vi "Example1.vi"() -> (0 "error out":errorcluster)   [LabVIEW 2020, in "Clippy.lvclass"]
uses:
  Clippy.lvclass
  AnimationTypes.ctl
panel:
  in  "Question":string
  out "Answer":string
  out "Picture":picture
  in  "Animate":bool
  in  "Animation":T1
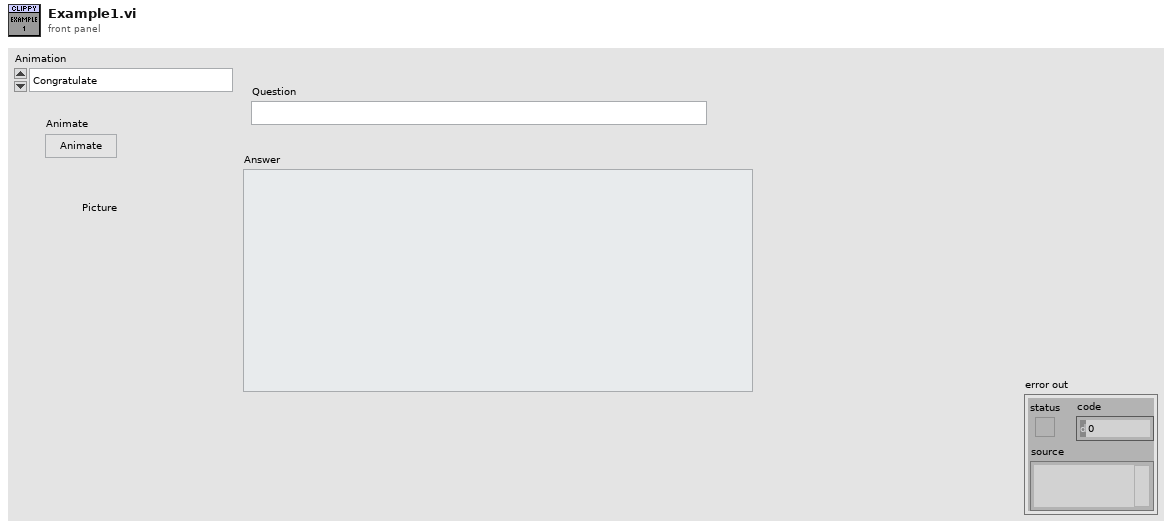
[diagram p1: front panel]
types:
  T1 = typedef "Clippy.lvclass/AnimationTypes.ctl" = enum16{"Congratulate", "LookRight", "SendMail", "Thinking", "Explain", "IdleRopePile", "IdleAtom", "Print", "Hide", "GetAttention", "Save", "GetTechy", "GestureUp", "Idle1_1", "Processing", "Alert", "LookUpRight", "IdleSideToSide", "GoodBye", "LookLeft", "IdleHeadScratch", "LookUpLeft", "CheckingSomething", "Hearing_1", "GetWizardy", "IdleFingerTap", "GestureLeft", "Wave", "GestureRight", "Writing", "IdleSnooze", "LookDownRight", "GetArtsy", "Show", "LookDown", "Searching", "EmptyTrash", "Greeting", "LookUp", "GestureDown", "RestPose", "IdleEyeBrowRaise", "LookDownLeft"}
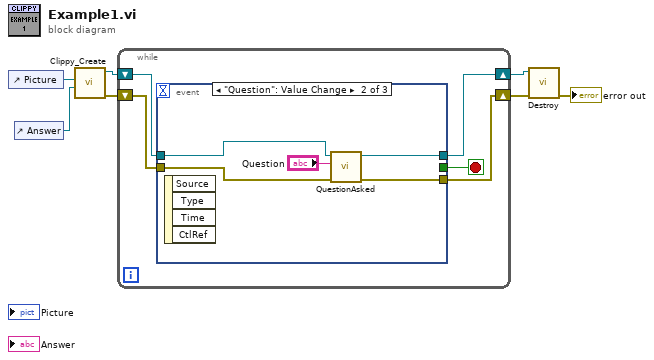
[diagram p0: block diagram]
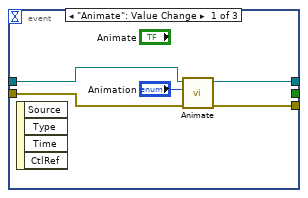
[diagram p2: hidden frame]
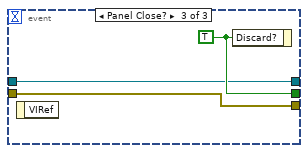
[diagram p3: hidden frame]
diagram:
  n1 = control-ref of="Picture"() -> (w2:refnum<vi>)
  n2 = control-ref of="Answer"() -> (w1:refnum<vi>)
  n3 = call "Clippy_Create.vi"("AnswerRef"=w1, "ClippyPictureRef"=w2) -> ("error out"=w7:errorcluster, "reference out"=w6:refnum<class "Clippy.lvclass">)  [unwired: 8 in]
  n4 = while {
    shift-right: [w10] -> w5
    shift-left: w7 -> [w12]
    shift-right: [w9] -> w4
    shift-left: w6 -> [w11]
    stop <- w8 stop-if-true
    n5 = event shown="[1] \"Question\": Value Change" {
      selector: _ -> [_ _ _]
      dyn-events: _ -> [_ _ _]
      timeout: _ -> [_ _ _]
      tunnel: w12 -> [w17 w21 w23]
      tunnel: w11 -> [w16 w22 w24]
      tunnel: [w15 w18 w23] -> w10
      tunnel: [w14 w19 w24] -> w9
      tunnel: [_ _ w25] -> w8
      event "Animate": Value Change {
        n6 = event-data() -> ()  [unwired: 1 in, 4 out]
        n7 = call-dynamic "Animate.vi"("Error In"=w17, "Animation"="Animation", "reference in"=w16) -> ("Error Out"=w15:errorcluster, "reference out"=w14:refnum<class "Clippy.lvclass">)  [unwired: 7 in]
      }
      event "Question": Value Change {
        n8 = event-data() -> ()  [unwired: 1 in, 4 out]
        n9 = call-dynamic "QuestionAsked.vi"("Error In"=w21, "Question"="Question", "reference in"=w22) -> ("Error Out"=w18:errorcluster, "reference out"=w19:refnum<class "Clippy.lvclass">)  [unwired: 7 in]
      }
      event Panel Close? {
        w25 = TRUE ("Discard?")
        n10 = event-data() -> ()  [unwired: 1 in, 1 out]
        n11 = event-data("Discard?"=w25) -> ()  [unwired: 1 in, 1 out]
      }
    }
  }
  n12 = call-dynamic "Destroy.vi"("error in (no error)"=w5, "reference in"=w4) -> ("error out"=→"error out":errorcluster)  [unwired: 8 in, 1 out]
